vi "Concatenate Composite String.vi"(11 "Array":string[](array[string])) -> (3 "String":string)   [LabVIEW 2017]
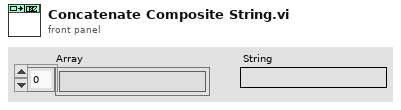
[diagram p1: front panel]
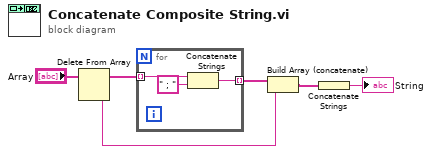
[diagram p0: block diagram]
diagram:
  n1 = Delete From Array(array="Array") -> (deleted portion=w3:string, array with subset deleted=w4:string[])  [unwired: 2 in]
  n2 = for {
    tunnel: [w8] -> w5 mode=indexing
    tunnel: w4 -> [w7] mode=indexing
    n3 = Concatenate Strings(w7, " ; " ("string")) -> (w8:string)
  }
  n4 = Build Array (concatenate)(w5, w3) -> (w2:string[])
  n5 = Concatenate Strings(w2) -> (→"String":string)
